vi "Print.vi"(0 "object in":refnum<class "Tree.lvclass">, 5 "Error In":errorcluster) -> (14 "object out":refnum<class "Tree.lvclass">, 16 "TreeString":string, 19 "Error Out":errorcluster)   [LabVIEW 2024, in "Tree.lvclass"]
uses:
  Tree.lvclass
  Tree.lvclass/Tree.ctl
  Node_class/Node.lvclass
panel:
  # "Connector Pane"
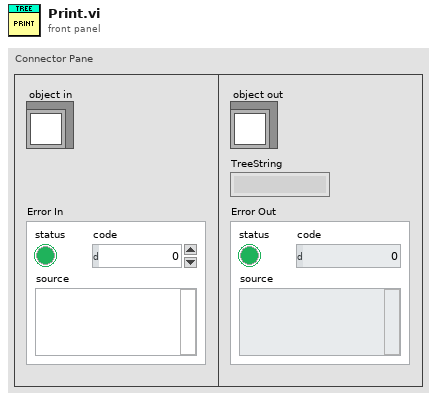
[diagram p1: front panel]
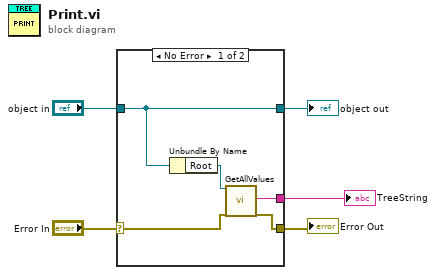
[diagram p0: block diagram]
diagram:
  n1 = case shown="No Error" "Error In" {
    selector: "Error In" -> [w8 w12]
    tunnel: [w7 w12] -> w4
    tunnel: [w10 w11] -> w2
    tunnel: "object in" -> [w10 w11]
    tunnel: [w6 _] -> w1
    frame No Error {
      n2 = Unbundle By Name(w10) -> ("Root"=w9:refnum<class "Node.lvclass">)
      n3 = call-dynamic "GetAllValues.vi"("object in"=w9, "Error In"=w8) -> ("Values"=w6:string, "Error Out"=w7:errorcluster)  [unwired: 15 in, 1 out]
    }
    frame Error {
    }
  }
  "Error Out" <- w4
  "object out" <- w2
  "TreeString" <- w1
